vi "Global.vi"() -> ()   [LabVIEW 2015, in "AIT 664 Custom Device.lvlib"]
uses:
  AIT 664 Custom Device.lvlib
panel:
  in  "Force hex Regenerate?":string="ForceHexRegen"
  in  "Licensed?":string="Licensed?"
  in  "Rx Message Ports Buffer Depth":string="Rx Message Ports Buffer Depth"
  in  "Rx Message Ports Port Rate (ms)":string="Rx Message Ports Port Rate (ms)"
  in  "Tx Message Ports Port Rate (ms)":string="Tx Message Ports Port Rate (ms)"
  in  "Main Page - VISA Address":string="Main Page - VISA Address"
  in  "Serial#":string="Serial#"
  in  "LicenseKey":string="LicenseKey"
  in  "AppLicense?":string="AppLicense?"
  in  "Tx Message Ports Destination UDP Port":string="Tx Message Ports Destination UDP Port"
  in  "Tx Message Ports Destination IP Address":string="Tx Message Ports Destination IP Address"
  in  "Tx Message Ports Source UDP Port":string="Tx Message Ports Source UDP Port"
  in  "Tx Message Ports Source IP Address":string="Tx Message Ports Source IP Address"
  in  "Rx Message Ports Destination UDP Port":string="Rx Message Ports Destination UDP Port"
  in  "Rx Message Ports Destination IP Address":string="Rx Message Ports Destination IP Address"
  in  "Rx Message Ports Source UDP Port":string="Rx Message Ports Source UDP Port"
  in  "Rx Message Ports Source IP Address":string="Rx Message Ports Source IP Address"
  in  "Rx Message Ports Sampling Type":string="Rx Message Ports Sampling Type"
  in  "Rx Message Ports Port Id":string="Rx Message Ports Port Id"
  in  "Input VL ID":string="Input VL ID"
  in  "Rx Message Ports Page GUID":string="85638AB9-73EA-4DD0-AE5B-CB4846ED525C"
  in  "Input VL Page GUID":string="213DE7A6-AD2E-4100-AAE2-F7F57146E2E9"
  in  "Tx Message Ports Sampling Type":string="Tx Message Ports Sampling Type"
  in  "Tx Message Ports Port Id":string="Tx Message Ports Port Id"
  in  "Tx Message Ports Page GUID":string="3F045D4F-17C3-4390-885C-937226A99FBD"
  in  "Output VL Page GUID":string="3935F3D2-468E-4B98-8B71-6F9ECDCE061D"
  in  "Output VL ID":string="Output VL ID"
  in  "End System Id":string="End System Id"
  in  "End System MAC Address":string="End System MAC Address"
  in  "MACAddress":string="MacAddress"
  in  "RTReadRate":string="BMReadRate"
  in  "Bus Monitor Msg Page GUID":string="9E1E077C-FA18-4FB1-8BDB-BA90D33E7B4A"
  in  "Remote Terminal Msg Page GUID":string="9E1E077C-FA18-4FB1-8BDB-BA90D33E7B4A"
  in  "Default Word":string="Default Word"
  in  "First Byte":string="First Byte"
  in  "Default Message Buffer Data":string="Default Message Buffer Data"
  in  "Message Buffer ID":string="Message Buffer ID"
  in  "RT Sub Address":string="RT Sub Address"
  in  "RT Address":string="RT Address"
  in  "Tx-Rx":string="Tx-Rx"
  in  "Message":string="Message"
  in  "RTName":string="Remote Terminals"
  in  "BMReadRate":string="BMReadRate"
  in  "BMName":string="Bus Monitor"
  in  "Message Parm Page GUID":string="68590DF2-265A-465B-BAB5-5ABE6CADE670"
  in  "Bus Controller Msg Page GUID":string="9E1E077C-FA18-4FB1-8BDB-BA90D33E7B4A"
  in  "BCParmName":string="BCMsgName"
  in  "BCMsgName":string="BCMsgName"
  in  "BCReadRate":string="BCReadRate"
  in  "Remote Termial Page GUID":string="0FC95884-141B-4A44-8C18-0C390E7B660A"
  in  "Bus Monitor Page GUID":string="779AC30D-0C9D-4D37-8E33-9253C541ED25"
  in  "End System Page GUID":string="2F575A5F-A4B6-4631-93A8-0AFA2722625C"
  in  "Bus Page GUID":string="DFEB7A51-36C0-42EF-8365-869E1AF267D7"
  in  "BCEnabled":string="BCEnabled"
  in  "BCName":string="Bus Controller"
  in  "BusNumber":string="BusNumber"
  in  "BusName":string="BusName"
  in  "ScaleOffset":string="ScaleOffset"
  in  "ScaleFac":string="ScaleFac"
  in  "Signed?":string="Signed?"
  in  "DBHash":string="DBHash"
  in  "MainDisabled":string="997C1B95-6D68-4D05-AFF2-98E404014BA2"
  in  "MainEnabled":string="4AA0FB30-DC4B-4C4E-8EA3-24E23807ABE5"
  in  "Static Chan GUID":string="C9C40DCC-9164-491A-ABAD-09896E38B425"
  in  "Default Value":string="Default Value"
  in  "NetworkSpeed":string="NetworSpeed"
  in  "Status Section GUID":string="F068105C-6F57-422F-81C9-D1E870E3340F"
  in  "Num Bits":string="Num Bits"
  in  "Win File Path":string="Win File Path"
  in  "Start Bit":string="Start Bit"
  # "NOTE: in the event other port types are implemented one would need new pages for them, \nthey do not have all of the same settings as the UDP ports"
  # "Output VL Page Items"
  # "Input VL Page Items"
  # "BC Parameter Page Items"
  # "Main Page Items"
  # "End System Page Items"
  # "Tx Message Ports Page Items"
  # "Rx Message Ports Page Items"
  # "Bus Page Items"
  # "BC Page Items"
  # "BC Msg Page Items"
  # "Section for Acyclic"
  # "Load/Referesh Database"
  # "BM Page Items"
  # "New"
  # "Old"
  # "Run Time Menu Item - Separator"
  # "7755077A-1485-13A6-5674A23FB86277FF"
  # "C4F6D306-C3D2-477F-8B0F-4F0FF7C0D36D"
  # "Run Time Menu Item - Disable"
  # "24B063C9-F831-AFAE-44CD-E299CAF12166"
  # "4BD42C26-0AA1-42C2-86E5-FB8DBEEA74AE"
  # "RT Page Items"
  # "Main Enabled"
  # "961BA415-D612-25DB-1EE4-93AC9399C9B8"
  # "9F0087A5-0D3D-41AC-84E7-59462FEFDFC4"
  # "D875045B-F708-417A-8922-E756FC4B70ED"
  # "Main Disabled"
  # "C84F327B-5F00-A71A-4A47-A7C0FE0BF79D"
  # "Static Chan"
  # "D9567732-A0D4-4249-9D7D-90741D022DA7"
  # "620FF26C-B46F-A798-9FE7-99E7CBCC898B"
  # "Status Section"
  # "40A8AAAE-6936-1961-F317-B9DADC611A49"
  # "2ECB6C91-3CC4-4FDF-AD6F-FA2D8CDB197F"
  # "GUIDS"
  # "Changed"
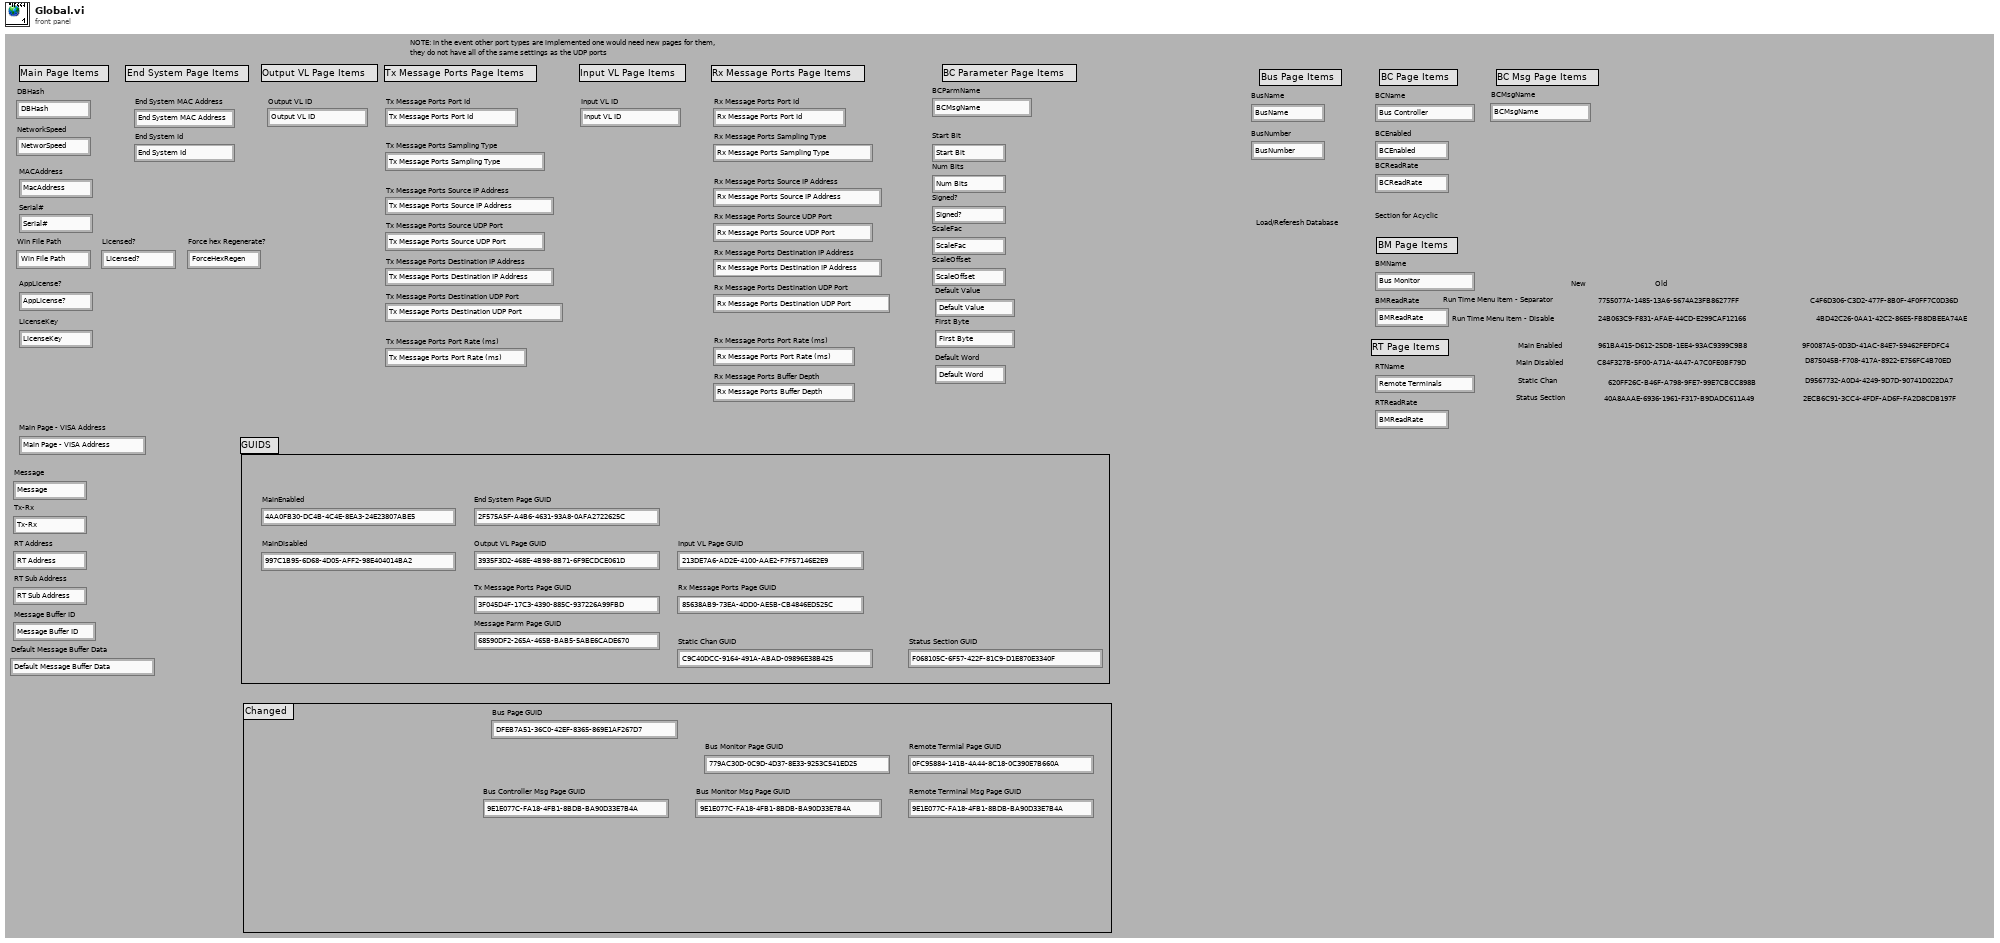
[diagram p1: front panel]
diagram:
